vi "保存mes.vi"(7 "温度instance":refnum<class "Modbus Master.lvclass">, 11 "参数值":T1(array[cluster])) -> (0 "已保存?":bool, 2 "进站OK?":bool)   [LabVIEW 2020]
uses:
  <vilib>/NI/Modbus Library/API/Master/Modbus Master.lvclass
  Global.vi
  <vilib>/Utility/file.llb/Write Delimited Spreadsheet (string).vi
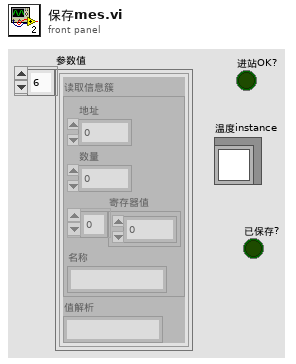
[diagram p1: front panel]
types:
  T1 = cluster{"读取信息簇":cluster{"地址":u16, "数量":u16, "寄存器值":u16[], "名称":string}, "值解析":string}[]
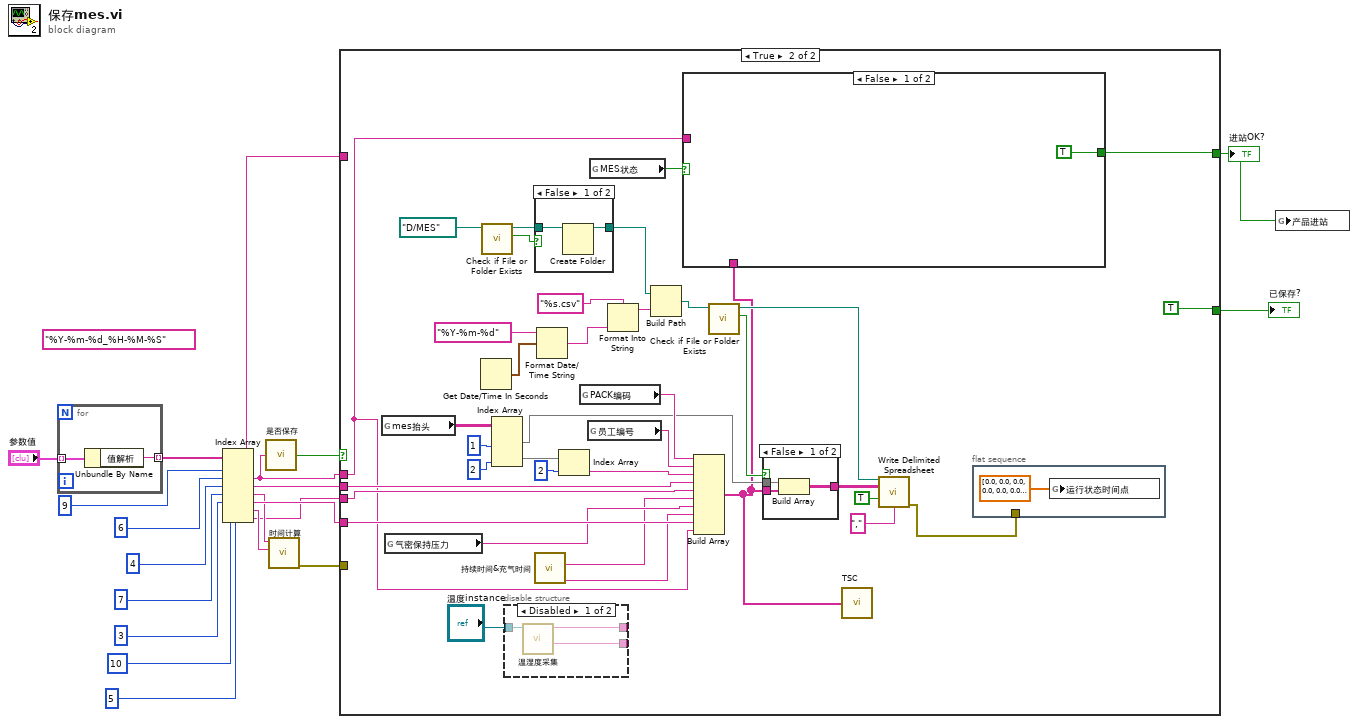
[diagram p0: block diagram]
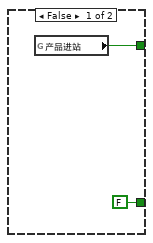
[diagram p2: hidden frame]
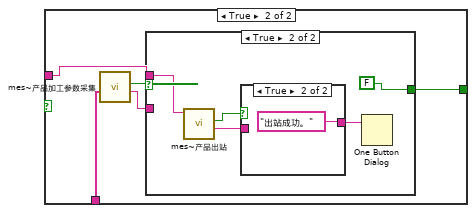
[diagram p4: hidden frame]
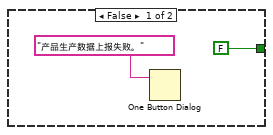
[diagram p5: hidden frame]
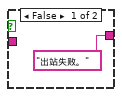
[diagram p6: hidden frame]
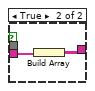
[diagram p7: hidden frame]
diagram:
  (unwired) "%Y-%m-%d_%H-%M-%S" ("时间格式字符串(%c)")
  n1 = for {
    tunnel: "参数值" -> [w22] mode=indexing
    tunnel: [w21] -> w19 mode=indexing
    n2 = Unbundle By Name(w22) -> ("值解析"=w21:string)
  }
  n3 = Index Array(array=w19, index #1=9 ("索引"), index #2=6 ("索引"), index #3=4 ("索引"), index #4=7 ("索引"), index #5=3 ("索引"), index #6=10 ("索引"), index #7=5 ("索引")) -> (element #1=w5:string, element #2=w14:string, element #3=w13:string, element #4=w9:string, element #5=w12:string, element #6=w8:string, element #7=w2:string)
  n4 = call "是否保存.vi"("测试结果"=w14) -> ("保存"=w11:bool)
  n5 = call "时间计算.vi"("运行状态"=w8, "实时压力"=w9) -> ("错误常量out"=w7:errorcluster)  [unwired: 9 in]
  n6 = case shown="True" w11 {
    tunnel: w14 -> [_ w27]
    tunnel: w13 -> [_ w48]
    tunnel: w2 -> [_ w47]
    tunnel: w12 -> [_ w46]
    tunnel: w7 -> [_ _]
    tunnel: w5 -> [_ _]
    tunnel: [w24 w30] -> w4
    tunnel: [FALSE TRUE] -> w1
    frame False {
      n7 = global read "Global.vi" "产品进站"() -> (w24:bool)
    }
    frame True {
      n8 = global read "Global.vi" "mes抬头"() -> (w56:string[][])
      n9 = global read "Global.vi" "气密保持压力"() -> (w34:string)
      n10 = Get Date/Time In Seconds() -> (seconds since 1Jan1904=w60:timestamp)
      n11 = call <vilib>:"Check if File or Folder Exists.vi"("path"=path "D:/MES" ("路径")) -> ("file or folder exists?"=w42:bool, "dup path"=w41:path)  [unwired: 8 in, 1 out]
      n12 = Index Array(array=w56, index (col) #1=1 ("禁用的索引 (列)"), index (col) #2=2 ("禁用的索引 (列)")) -> (element #1=w45:string[], element #2=w53:string[])  [unwired: 2 in]
      n13 = disable-structure shown="Disabled" {
        disable-tunnel: "温度instance" -> [w64 _]
        disable-tunnel: [w63 _] -> _
        disable-tunnel: [w62 _] -> _
        frame Disabled {
          n14 = call "温湿度采集.vi"("Modbus Master输入"=w64) -> ("温度"=w62:string, "湿度"=w63:string)  [unwired: 9 in]
        }
        frame Enabled {
        }
      }
      n15 = case shown="False" w42 {
        tunnel: w41 -> [w87 w88]
        tunnel: [w86 w88] -> w38
        frame False {
          n16 = Create Folder(path (use dialog)=w87) -> (created path=w86:path)  [unwired: 2 in, 2 out]
        }
        frame True {
        }
      }
      n17 = call "持续时间&充气时间.vi"() -> ("气密保持压力持续时间"=w31:string, "气密充气时间"=w32:string)  [unwired: 10 in]
      n18 = Format Date/Time String(time format string (%c)="%Y-%m-%d" ("时间格式字符串(%c)"), seconds (now)=w60) -> (date/time string=w58:string)  [unwired: 1 in]
      n19 = Index Array(array=w53, index=2 ("索引")) -> (element=w49:string)
      n20 = global read "Global.vi" "PACK编码"() -> (w51:string)
      n21 = global read "Global.vi" "员工编号"() -> (w50:string)
      n22 = global read "Global.vi" "MES状态"() -> (w29:bool)
      n23 = Format Into String(format string="%s.csv" ("格式字符串"), w58) -> (resulting string=w57:string)  [unwired: 2 in, 1 out]
      n24 = Build Path(base path=w38, name or relative path=w57) -> (appended path=w37:path)
      n25 = Build Array(w51, w50, w49, w48, w47, w32, w34, w31, w46, w27) -> (w26:string[])
      n26 = case shown="False" w29 {
        tunnel: w27 -> [_ w70]
        tunnel: w26 -> [_ w69]
        tunnel: [TRUE w66] -> w30
        frame False {
        }
        frame True {
          n27 = call "mes~产品加工参数采集.vi"("采集项"=w69) -> ("ErrorMessage"=w67:string, "加工参数采集成功"=w68:bool)  [unwired: 8 in, 1 out]
          n28 = case shown="True" w68 {
            tunnel: w70 -> [_ w77]
            tunnel: w67 -> [_ _]
            tunnel: [FALSE FALSE] -> w66
            frame False {
              n29 = One Button Dialog(message="产品生产数据上报失败。") -> ()  [unwired: 1 in, 1 out]
            }
            frame True {
              n30 = call "mes~产品出站.vi"("测试结果"=w77) -> ("ErrorMessage"=w75:string, "出站成功"=w76:bool)  [unwired: 8 in, 1 out]
              n31 = case shown="True" w76 {
                tunnel: w75 -> [_ _]
                tunnel: ["出站失败。" "出站成功。"] -> w74
                frame False {
                }
                frame True {
                }
              }
              n32 = One Button Dialog(message=w74) -> ()  [unwired: 1 in, 1 out]
            }
          }
        }
      }
      n33 = call <vilib>:"Check if File or Folder Exists.vi"("path"=w37) -> ("file or folder exists?"=w36:bool, "dup path"=w35:path)  [unwired: 8 in, 1 out]
      n34 = case shown="False" w36 {
        tunnel: w45 -> [w83 _]
        tunnel: w26 -> [w82 w85]
        tunnel: [w81 w84] -> w44
        frame False {
          n35 = Build Array(w83, w82) -> (w81:string[][])
        }
        frame True {
          n36 = Build Array(w85) -> (w84:string[][])
        }
      }
      n37 = call "TSC.vi"("参数"=w26) -> ()
      n38 = call-poly <vilib>:"Write Delimited Spreadsheet.vi"("file path (dialog if empty)"=w35, "2D data"=w44, "append to file? (new file:F)"=TRUE ("append to file? (F)"), "delimiter (\\t)"="," ("delimiter (\\t)")) -> ("error out"=w33:errorcluster)  [unwired: 10 in, 1 out]
      n39 = flat-sequence {
        tunnel: w33 -> [_]
        frame #0 {
          n40 = global write "Global.vi" "运行状态时间点"(dbl[] [0.0, 0.0, 0.0, 0.0, 0.0, 0.0, 0.0, 0.0, 0.0] ("运行状态时间点")) -> ()
        }
      }
    }
  }
  "进站OK?" <- w4
  "已保存?" <- w1
  n41 = global write "Global.vi" "产品进站"(w4) -> ()
